vi "Program Scene.vi"(8 "error in (no error)":errorcluster, 11 "RGetCurrentProgramScene in":refnum<class "RGetCurrentProgramScene.lvclass">) -> (0 "error out":errorcluster, 2 "Program Scene":string, 3 "RGetCurrentProgramScene out":refnum<class "RGetCurrentProgramScene.lvclass">)   [LabVIEW 2022 SP3, in "obs-websocket-lv.lvlib" / "RGetCurrentProgramScene.lvclass"]
uses:
  RGetCurrentProgramScene.lvclass
  RGetCurrentProgramScene.lvclass/RGetCurrentProgramScene.ctl
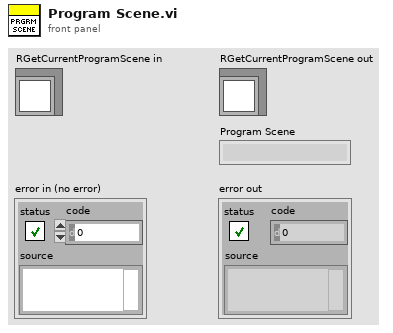
[diagram p1: front panel]
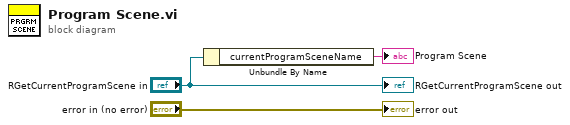
[diagram p0: block diagram]
diagram:
  n1 = Unbundle By Name("RGetCurrentProgramScene in") -> ("currentProgramSceneName"=→"Program Scene":string)
  "error out" <- "error in (no error)"
  "RGetCurrentProgramScene out" <- "RGetCurrentProgramScene in"
